vi "device_close.vi"(8 "error in":errorcluster, 11 "New Focus Model 8742.lvclass":refnum<class "New Focus Model 8742.lvclass">) -> (0 "error out":errorcluster)   [LabVIEW 2020, in "New Focus Model 8742.lvclass"]
uses:
  New Focus Model 8742.lvclass
  New Focus Model 8742.lvclass/New Focus Model 8742.ctl
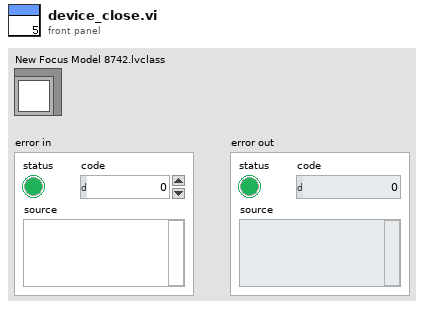
[diagram p1: front panel]
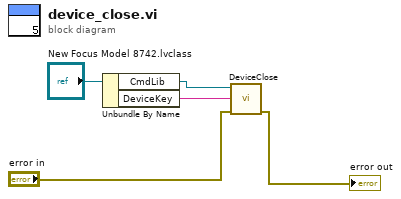
[diagram p0: block diagram]
diagram:
  n1 = Unbundle By Name("New Focus Model 8742.lvclass") -> ("CmdLib"=w4:refnum<k24>, "DeviceKey"=w3:string)
  n2 = call <instrlib>:"DeviceClose.vi"("error in (no error)"="error in", "DeviceKey In"=w3, "CmdLib In"=w4) -> ("error out"=→"error out":errorcluster)  [unwired: 2 in, 2 out]
